vi "Read Model Enqueuer.vi"(11 "IViewModel In":refnum<class "IViewModel.lvclass">) -> (2 "Model Enqueuer":refnum<class "Message Enqueuer.lvclass">)   [LabVIEW 2017, in "IViewModel.lvlib" / "IViewModel.lvclass"]
doc: "Use Read Root Model Enqueuer\n(Same thing, clearer name)"
uses:
  IViewModel.lvclass
  <vilib>/ActorFramework/Message Enqueuer/Message Enqueuer.lvclass
  IViewModel.lvclass/IViewModel.ctl
panel:
  # "Use Read Root Model Enqueuer\n(Same thing, clearer name)"
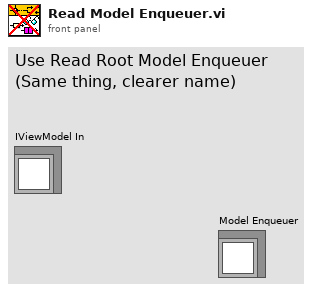
[diagram p1: front panel]
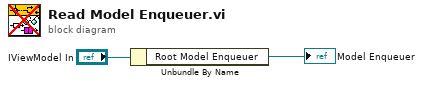
[diagram p0: block diagram]
diagram:
  n1 = Unbundle By Name("IViewModel In") -> ("Root Model Enqueuer"=→"Model Enqueuer":refnum<class "Message Enqueuer.lvclass">)
